vi "公式复合写入.vi"(8 "公式":cluster{"X^2":dbl, "X":dbl, "b":dbl}, 9 "量程下拉列表":enum16{"低量程", "高量程"}(ring), 10 "测量模式下拉列表":enum16{"水样测量", "零点核查", "跨度核查", "标样核查", "加标回收"}(ring), 11 "参数下拉列表":u16(ring) items=["总氮"=2, "总磷"=1, "磷酸盐"=4]) -> (3 "模型复制":T1)   [LabVIEW 2016, in "斯坦道总氮.lvlib"]
uses:
  <vilib>/Utility/miscctls.llb/LVPointTypeDef.ctl
panel:
  out "连接的字符串":string
  in  "取消":bool
  in  "确认":bool
  in  "加标回收":bool
  in  "标样核查":bool
  in  "跨度核查":bool
  in  "空白核查":bool
  in  "水样测量":bool=TRUE
  # "请选择要写入的参数"
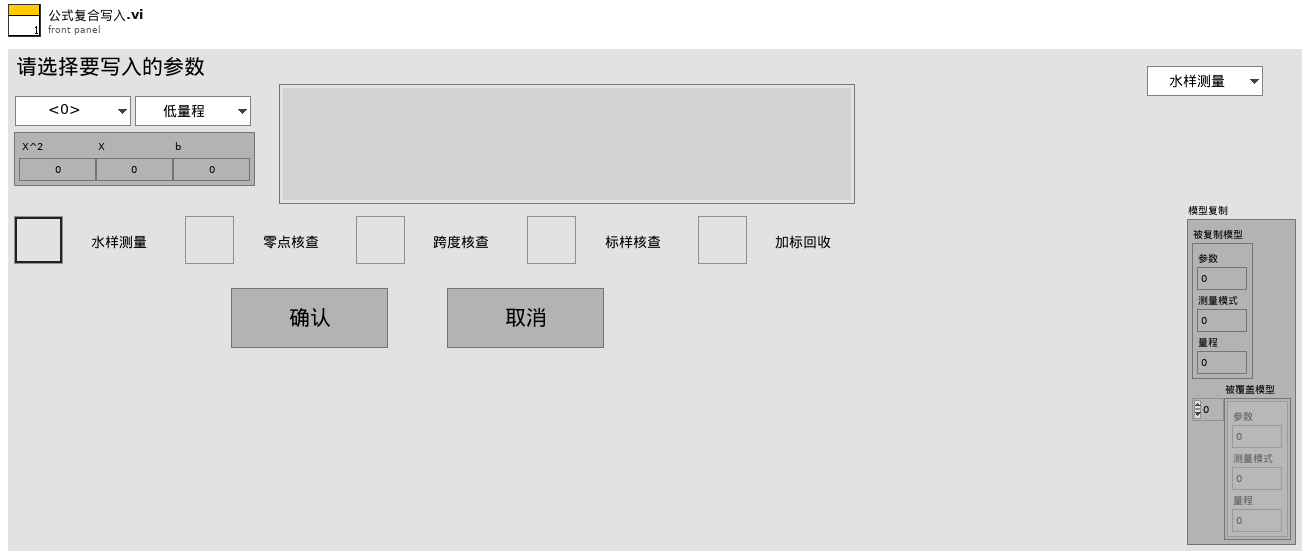
[diagram p1: front panel]
types:
  T1 = cluster{"被复制模型":cluster{"参数":u8, "测量模式":u8, "量程":u8}, "被覆盖模型":cluster{"参数":u8, "测量模式":u8, "量程":u8}[]}
  T2 = typedef "LVPointTypeDef.ctl" = cluster{"Horizontal":i16, "Vertical":i16}
  T3 = typedef "LVStringsAndValuesArrayTypeDef_U16.ctl" = cluster{"String":string, "Value":u16}[]
  T4 = cluster{"参数下拉列表":u16, "测量模式":enum16{"水样测量", "零点核查", "跨度核查", "标样核查", "加标回收"}, "量程下拉列表":enum16{"低量程", "高量程"}}
  T5 = cluster{"参数下拉列表":u16, "测量模式":enum16{"水样测量", "零点核查", "跨度核查", "标样核查", "加标回收"}, "量程下拉列表":enum16{"低量程", "高量程"}}[]
  T6 = cluster{"测量量程":dbl, "测量精度":dbl, "测量间隔":dbl, "消解温度":dbl, "消解时长":dbl, "空白校准时间":timestamp, "曲线截距":dbl, "曲线斜率":dbl, "测量检出限":dbl, "测量信号值":dbl, "线性相关系数":dbl, "二次多项式系数":dbl, "标样校准时间":timestamp, "稀释倍数":dbl, "三项式系数":dbl, "空白标定系数":dbl, "量程系数":dbl, "F0/ORPA":dbl, "F1/ORPB":dbl, "F2/ORPK":dbl, "F3":dbl, "F4":dbl, "F5":dbl, "F6":dbl, "F7":dbl, "X0/滴定数":dbl, "量程":dbl}
  T7 = cluster{"参数下拉列表":u16, "测量模式下拉列表":enum16{"水样测量", "零点核查", "跨度核查", "标样核查", "加标回收"}, "量程下拉列表":enum16{"低量程", "高量程"}}
  T8 = cluster{cluster{"参数下拉列表":u16, "测量模式下拉列表":enum16{"水样测量", "零点核查", "跨度核查", "标样核查", "加标回收"}, "量程下拉列表":enum16{"低量程", "高量程"}}, cluster{"参数下拉列表":u16, "测量模式下拉列表":enum16{"水样测量", "零点核查", "跨度核查", "标样核查", "加标回收"}, "量程下拉列表":enum16{"低量程", "高量程"}}[]}
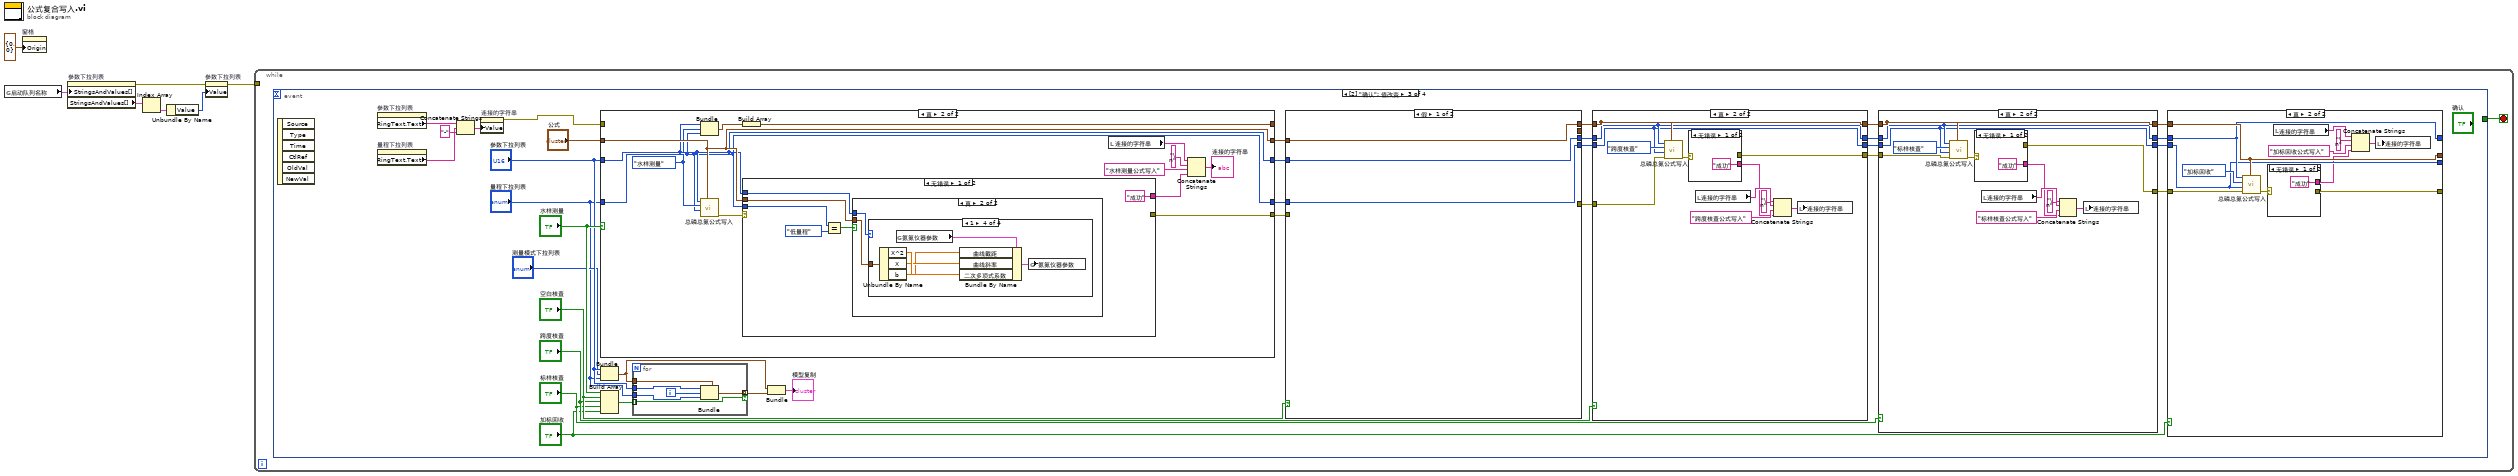
[diagram p0: block diagram]
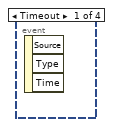
[diagram p2: hidden frame]
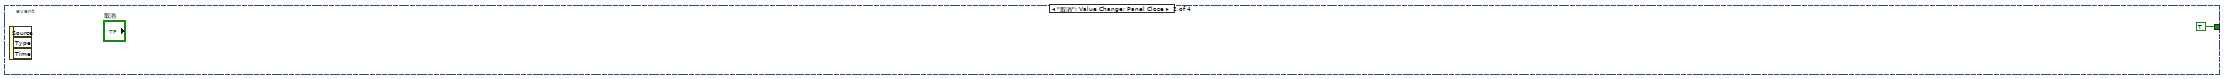
[diagram p3: hidden frame]
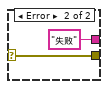
[diagram p5: hidden frame]
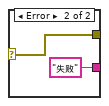
[diagram p7: hidden frame]
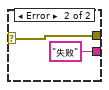
[diagram p9: hidden frame]
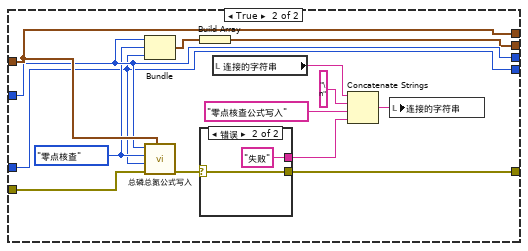
[diagram p10: hidden frame]
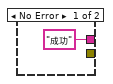
[diagram p11: hidden frame]
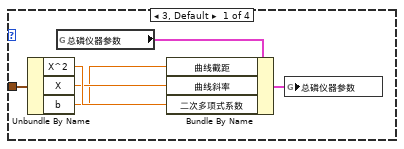
[diagram p14: hidden frame]
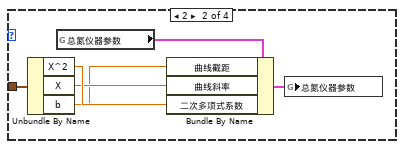
[diagram p15: hidden frame]
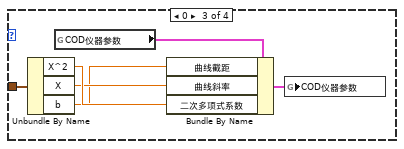
[diagram p16: hidden frame]
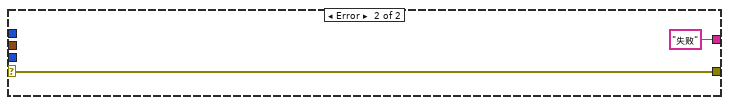
[diagram p17: hidden frame]
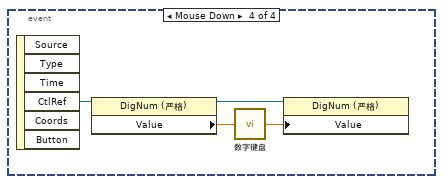
[diagram p18: hidden frame]
diagram:
  n1 = global read "总磷总氮断电保存全局变量.vi" "启动队列名称"() -> (w6:cluster{"String":string, "Value":u16}[])
  n2 = property on="窗格" class="Pane"("Origin"=T2 {"Horizontal"=0, "Vertical"=0} ("原点")) -> ()  [unwired: 2 in, 2 out]
  n3 = property on="参数下拉列表" class="Ring (严格)"("StringsAndValues[]"=w6) -> (error out=w5:errorcluster, "StringsAndValues[]"=w3:T3)  [unwired: 2 in, 1 out]
  n4 = Index Array(array=w3) -> (element=w2:cluster{"String":string, "Value":u16})  [unwired: 1 in]
  n5 = Unbundle By Name(w2) -> ("Value"=w1:u16)
  n6 = property on="参数下拉列表" class="Ring (严格)"(error in=w5, "Value"=w1) -> (error out=w4:errorcluster)  [unwired: 1 in, 1 out]
  n7 = while {
    tunnel: w4 -> [_]
    stop <- w8 stop-if-true
    n8 = event shown="[2] \"确认\": 值改变" {
      selector: _ -> [_ _ _ _]
      dyn-events: _ -> [_ _ _ _]
      timeout: _ -> [_ _ _ _]
      tunnel: [_ TRUE _ _] -> w8
      event Timeout {
        n9 = event-data() -> ()  [unwired: 1 in, 3 out]
      }
      event "取消": Value Change; Panel Close {
        n10 = event-data() -> ()  [unwired: 1 in, 3 out]
      }
      event "确认": Value Change {
        n11 = event-data() -> ()  [unwired: 1 in, 6 out]
        n12 = property on="参数下拉列表" class="Ring (严格)"() -> ("RingText.Text"=w24:string)  [unwired: 2 in, 2 out]
        n13 = property on="量程下拉列表" class="Enum (严格)"() -> ("RingText.Text"=w23:string)  [unwired: 2 in, 2 out]
        n14 = Concatenate Strings(w24, "-" ("字符串"), w23) -> (w25:string)
        n15 = property on="连接的字符串" class="Str"("Value"=w25) -> (error out=w26:errorcluster)  [unwired: 2 in, 1 out]
        n16 = case shown="真" "水样测量" {
          tunnel: "公式" -> [w126 w132]
          tunnel: "参数下拉列表" -> [w125 w131]
          tunnel: "量程下拉列表" -> [w124 w129]
          tunnel: [w126 w132] -> w42
          tunnel: [w125 w131] -> w41
          tunnel: [w124 w129] -> w40
          tunnel: [_ w138] -> w28
          tunnel: w26 -> [_ _]
          tunnel: [_ w127] -> _
          frame False {
          }
          frame True {
            w130 = enum16{"水样测量", "零点核查", "跨度核查", "标样核查", "加标回收"}."水样测量" ("测量模式")
            n17 = Bundle("参数下拉列表"=w131, "测量模式"=w130, "量程下拉列表"=w129) -> (w128:T4)  [unwired: 1 in]
            n18 = call "总磷总氮公式写入.vi"("公式"=w132, "量程"=w129, "测量模式"=w130, "测量参数"=w131) -> ("error out"=w139:errorcluster)  [unwired: 7 in]
            n19 = Build Array(w128) -> (w127:T5)
            n20 = case shown="无错误" w139 {
              selector: w139 -> [_ w173]
              tunnel: [_ w173] -> w138
              tunnel: ["成功" "失败"] -> w137
              tunnel: w129 -> [w144 _]
              tunnel: w131 -> [w141 _]
              tunnel: w132 -> [w140 _]
              frame No Error {
                n21 = Equal?(x=w144, y=enum16{"低量程", "高量程"}."低量程") -> (x = y?=w142:bool)
                n22 = case shown="真" w142 {
                  tunnel: w141 -> [_ w147]
                  tunnel: w140 -> [_ w146]
                  frame False {
                  }
                  frame True {
                    n23 = case shown="1" w147 {
                      tunnel: w146 -> [w148 w154 w160 w166]
                      frame 3, Default {
                        n24 = Unbundle By Name(w148) -> ("X^2"=w151:dbl, "X"=w150:dbl, "b"=w149:dbl)
                        n25 = global read "总磷总氮断电保存全局变量.vi" "总磷仪器参数"() -> (w152:T6)
                        n26 = Bundle By Name(cluster=w152, "曲线截距"=w149, "曲线斜率"=w150, "二次多项式系数"=w151) -> (w153:T6)
                        n27 = global write "总磷总氮断电保存全局变量.vi" "总磷仪器参数"(w153) -> ()
                      }
                      frame 2 {
                        n28 = Unbundle By Name(w154) -> ("X^2"=w157:dbl, "X"=w156:dbl, "b"=w155:dbl)
                        n29 = global read "总磷总氮断电保存全局变量.vi" "总氮仪器参数"() -> (w158:T6)
                        n30 = Bundle By Name(cluster=w158, "曲线截距"=w155, "曲线斜率"=w156, "二次多项式系数"=w157) -> (w159:T6)
                        n31 = global write "总磷总氮断电保存全局变量.vi" "总氮仪器参数"(w159) -> ()
                      }
                      frame 0 {
                        n32 = Unbundle By Name(w160) -> ("X^2"=w163:dbl, "X"=w162:dbl, "b"=w161:dbl)
                        n33 = global read "总磷总氮断电保存全局变量.vi" "COD仪器参数"() -> (w164:T6)
                        n34 = Bundle By Name(cluster=w164, "曲线截距"=w161, "曲线斜率"=w162, "二次多项式系数"=w163) -> (w165:T6)
                        n35 = global write "总磷总氮断电保存全局变量.vi" "COD仪器参数"(w165) -> ()
                      }
                      frame 1 {
                        n36 = Unbundle By Name(w166) -> ("X^2"=w169:dbl, "X"=w168:dbl, "b"=w167:dbl)
                        n37 = global read "总磷总氮断电保存全局变量.vi" "氨氮仪器参数"() -> (w170:T6)
                        n38 = Bundle By Name(cluster=w170, "曲线截距"=w167, "曲线斜率"=w168, "二次多项式系数"=w169) -> (w171:T6)
                        n39 = global write "总磷总氮断电保存全局变量.vi" "氨氮仪器参数"(w171) -> ()
                      }
                    }
                  }
                }
              }
              frame Error {
              }
            }
            n40 = local read "连接的字符串"() -> (w134:string)
            n41 = Concatenate Strings(w134, "\n" ("字符串"), "水样测量公式写入", w137) -> (→"连接的字符串":string)
          }
        }
        n42 = Bundle("参数下拉列表"="参数下拉列表", "测量模式下拉列表"="测量模式下拉列表", "量程下拉列表"="量程下拉列表") -> (w12:T7)  [unwired: 1 in]
        n43 = Build Array("水样测量", "空白核查", "跨度核查", "标样核查", "加标回收") -> (w16:bool[])
        n44 = for {
          tunnel: w16 -> [w45] mode=indexing
          tunnel: "参数下拉列表" -> [w49]
          tunnel: "量程下拉列表" -> [w47]
          tunnel: [w46] -> w11 mode=indexing if=w45
          tunnel: w12 -> [w44]
          i -> [w48]
          n45 = Bundle(cluster=w44, "参数下拉列表"=w49, "测量模式下拉列表"=w48, "量程下拉列表"=w47) -> (w46:T7)
        }
        n46 = Bundle(w12, w11) -> (→"模型复制":T8)  [unwired: 1 in]
        n47 = case shown="假" "空白核查" {
          tunnel: w42 -> [w106 w120]
          tunnel: w41 -> [w105 w110]
          tunnel: w40 -> [w104 w108]
          tunnel: [_ w115] -> w39
          tunnel: [w106 w120] -> w38
          tunnel: [w105 w110] -> w37
          tunnel: [w104 w108] -> w36
          tunnel: w28 -> [_ w119]
          tunnel: [_ w107] -> _
          frame False {
          }
          frame True {
            w109 = enum16{"水样测量", "零点核查", "跨度核查", "标样核查", "加标回收"}."零点核查" ("测量模式")
            n48 = Bundle("参数下拉列表"=w110, "测量模式"=w109, "量程下拉列表"=w108) -> (w111:T4)  [unwired: 1 in]
            n49 = call "总磷总氮公式写入.vi"("公式"=w120, "error in (no error)"=w119, "量程"=w108, "测量模式"=w109, "测量参数"=w110) -> ("error out"=w116:errorcluster)  [unwired: 6 in]
            n50 = Build Array(w111) -> (w107:T5)
            n51 = case shown="错误" w116 {
              selector: w116 -> [_ w123]
              tunnel: [_ w123] -> w115
              tunnel: ["成功" "失败"] -> w117
              frame No Error {
              }
              frame Error {
              }
            }
            n52 = local read "连接的字符串"() -> (w114:string)
            n53 = Concatenate Strings(w114, "\n" ("字符串"), "零点核查公式写入", w117) -> (w112:string)
            n54 = local write "连接的字符串"(w112) -> ()
          }
        }
        n55 = case shown="真" "跨度核查" {
          tunnel: w38 -> [w88 w99]
          tunnel: w37 -> [w87 w98]
          tunnel: w36 -> [w86 w97]
          tunnel: [w88 w99] -> w35
          tunnel: [w87 w98] -> w33
          tunnel: [w86 w97] -> w32
          tunnel: w39 -> [_ w96]
          tunnel: [_ w89] -> w27
          frame False {
          }
          frame True {
            n56 = call "总磷总氮公式写入.vi"("公式"=w99, "error in (no error)"=w96, "量程"=w97, "测量模式"=enum16{"水样测量", "零点核查", "跨度核查", "标样核查", "加标回收"}."跨度核查", "测量参数"=w98) -> ("error out"=w90:errorcluster)  [unwired: 6 in]
            n57 = case shown="无错误" w90 {
              selector: w90 -> [_ w103]
              tunnel: [_ w103] -> w89
              tunnel: ["成功" "失败"] -> w91
              frame No Error {
              }
              frame Error {
              }
            }
            n58 = local read "连接的字符串"() -> (w93:string)
            n59 = Concatenate Strings(w93, "\n" ("字符串"), "跨度核查公式写入", w91) -> (w95:string)
            n60 = local write "连接的字符串"(w95) -> ()
          }
        }
        n61 = case shown="真" "标样核查" {
          tunnel: w35 -> [w70 w81]
          tunnel: w33 -> [w69 w80]
          tunnel: w32 -> [w68 w79]
          tunnel: [_ w71] -> w29
          tunnel: [w70 w81] -> w34
          tunnel: [w69 w80] -> w31
          tunnel: [w68 w79] -> w30
          tunnel: w27 -> [_ w78]
          frame False {
          }
          frame True {
            n62 = call "总磷总氮公式写入.vi"("公式"=w81, "error in (no error)"=w78, "量程"=w79, "测量模式"=enum16{"水样测量", "零点核查", "跨度核查", "标样核查", "加标回收"}."标样核查", "测量参数"=w80) -> ("error out"=w72:errorcluster)  [unwired: 6 in]
            n63 = case shown="无错误" w72 {
              selector: w72 -> [_ w85]
              tunnel: [_ w85] -> w71
              tunnel: ["成功" "失败"] -> w73
              frame No Error {
              }
              frame Error {
              }
            }
            n64 = local read "连接的字符串"() -> (w75:string)
            n65 = Concatenate Strings(w75, "\n" ("字符串"), "标样核查公式写入", w73) -> (w77:string)
            n66 = local write "连接的字符串"(w77) -> ()
          }
        }
        n67 = case shown="真" "加标回收" {
          tunnel: w34 -> [w52 w63]
          tunnel: w31 -> [w51 w62]
          tunnel: w30 -> [w50 w61]
          tunnel: [w52 w63] -> _
          tunnel: [w51 w62] -> _
          tunnel: [w50 w61] -> _
          tunnel: w29 -> [_ w60]
          tunnel: [_ w53] -> _
          frame False {
          }
          frame True {
            n68 = call "总磷总氮公式写入.vi"("公式"=w63, "error in (no error)"=w60, "量程"=w61, "测量模式"=enum16{"水样测量", "零点核查", "跨度核查", "标样核查", "加标回收"}."加标回收", "测量参数"=w62) -> ("error out"=w54:errorcluster)  [unwired: 6 in]
            n69 = case shown="无错误" w54 {
              selector: w54 -> [_ w67]
              tunnel: [_ w67] -> w53
              tunnel: ["成功" "失败"] -> w55
              frame No Error {
              }
              frame Error {
              }
            }
            n70 = local read "连接的字符串"() -> (w57:string)
            n71 = Concatenate Strings(w57, "\n" ("字符串"), "加标回收公式写入", w55) -> (w59:string)
            n72 = local write "连接的字符串"(w59) -> ()
          }
        }
      }
      event "公式.X^2", "公式.X", "公式.b": Mouse Down {
        n73 = event-data() -> ("CtlRef"=w177:refnum<vi>)  [unwired: 1 in, 5 out]
        n74 = property class="DigNum (严格)"(reference=w177) -> (reference out=w174:refnum<vi>, "Value"=w176:dbl)  [unwired: 1 in, 1 out]
        n75 = call "数字键盘.vi"("OldNumber"=w176) -> ("NewNumber"=w175:dbl)
        n76 = property class="DigNum (严格)"(reference=w174, "Value"=w175) -> ()  [unwired: 1 in, 2 out]
      }
    }
  }
